vi "solar Log.vi"(6 "Clear Error? (T)":bool=TRUE, 7 "Type (TLM)":enum8{"CMD", "TLM"}(ring)=enum."TLM", 8 "error in (no error)":errorcluster, 9 "DATA":variant, 10 "MSG":string, 11 "solar in":refnum<class "solar.lvclass">) -> (0 "error out":errorcluster, 3 "solar out":refnum<class "solar.lvclass">)   [LabVIEW 2018, in "solar.lvclass"]
doc: "This enqueues a SOLAR log message to the logging process. Set <b>Clear Error?</b> to true to clear the error."
uses:
  solar.lvclass
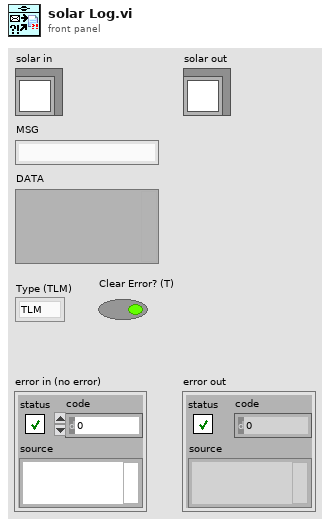
[diagram p1: front panel]
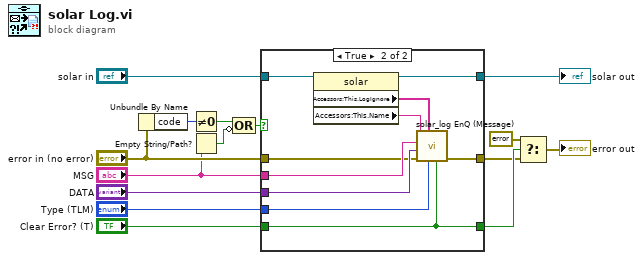
[diagram p0: block diagram]
diagram:
  n1 = Unbundle By Name("error in (no error)") -> ("code"=w8:i32)
  n2 = Not Equal To 0?(x=w8) -> (x != 0?=w7:bool)
  n3 = Empty String/Path?(string/path="MSG") -> (empty?=w6:bool)
  n4 = Compound Arithmetic op=OR(w7, invert w6) -> (w5:bool)
  n5 = case shown="True" w5 {
    tunnel: [w17 w28] -> w2
    tunnel: "DATA" -> [_ w27]
    tunnel: "Clear Error? (T)" -> [w16 w19]
    tunnel: "Type (TLM)" -> [_ w26]
    tunnel: "solar in" -> [w18 w23]
    tunnel: [w18 w22] -> w11
    tunnel: "MSG" -> [_ w21]
    tunnel: "error in (no error)" -> [w17 w20]
    tunnel: [w16 w19] -> w3
    frame False {
    }
    frame True {
      n6 = property class="solar"(reference=w23) -> (reference out=w22:refnum<class "solar.lvclass">, "Accessors:This.LogIgnore"=w24:string[], "Accessors:This.Name"=w25:string)  [unwired: 1 in, 1 out]
      n7 = call "solar_log EnQ (Message).vi"("Clear Error? (T)"=w19, "Type (CMD)"=w26, "LogIgnore"=w24, "error in (no error)"=w20, "DATA"=w27, "MSG"=w21, "Target"=w25) -> ("error out"=w28:errorcluster)  [unwired: 4 in]
    }
  }
  "solar out" <- w11
  n8 = Select(t=errorcluster {"status"=FALSE, "code"=0, "source"=""}, s=w3, f=w2) -> (s? t:f=→"error out":errorcluster)
